vi "外观.vi"(0 "Data In":T9={"启动"=FALSE, "控制命令"=enum."加标回收（启动采配水）", "测量参数"={"氨氮"=TRUE, "总磷"=TRUE, "总氮"=TRUE, "CODMn"=TRUE, "CODCr"=TRUE}} caption="数据输入", 2 "Display State In":T2={"配置信息"={"周期模式"=enum."不启用", "定点周期"={"启动命令"=0, "启动命令 2"=0, "启动命令 3"=0, "启动命令 4"=0, "启动命令 5"=0, "启动命令 6"=0, "启动命令 7"=0, "启动命令 8"=0, "启动命令 9"=0, "启动命令 10"=0, "启动命令 11"=0, "启动命令 12"=0, "启动命令 13"=0, "启动命令 14"=0, "启动命令 15"=0, "启动命令 16"=0, "启动命令 17"=0, "启动命令 18"=0, "启动命令 19"=0, "启动命令 20"=0, "启动命令 21"=0, "启动命令 22"=0, "启动命令 23"=0, "启动命令 24"=0}, "间隔启动"={"启动命令"=0, "启动间隔"=0.0, "启动次数"=0}, "测量参数"={"氨氮"=TRUE, "总磷"=TRUE, "总氮"=TRUE, "CODMn"=TRUE, "CODCr"=TRUE}}, "仪器运行状态"=FALSE, "启动次数"=0, "最近一次启动时间"=timestamp(0 s since 1904-01-01), "最近一次结束时间"=timestamp(0 s since 1904-01-01), "间隔计时"=0.0, "时间源"={"时间源选择"=enum."系统时间源", "外部时间源"=timestamp(0 s since 1904-01-01)}, "引用参数"="", "启用参数"={"氨氮"=TRUE, "总磷"=TRUE, "总氮"=TRUE, "CODMn"=TRUE, "CODCr"=FALSE}} caption="显示状态输入" {"配置信息"."间隔启动"."启动命令" items=["", "加标回收（启动采配水）", "加标回收（不启动采配水）", "水样测试（启动采配水）", "水样测试（不启动采配水）"]; "配置信息"."定点周期"."启动命令 24" items=["", "加标回收（启动采配水）", "加标回收（不启动采配水）", "水样测试（启动采配水）", "水样测试（不启动采配水）"]; "配置信息"."定点周期"."启动命令 23" items=["", "加标回收（启动采配水）", "加标回收（不启动采配水）", "水样测试（启动采配水）", "水样测试（不启动采配水）"]; "配置信息"."定点周期"."启动命令 22" items=["", "加标回收（启动采配水）", "加标回收（不启动采配水）", "水样测试（启动采配水）", "水样测试（不启动采配水）"]; "配置信息"."定点周期"."启动命令 21" items=["", "加标回收（启动采配水）", "加标回收（不启动采配水）", "水样测试（启动采配水）", "水样测试（不启动采配水）"]; "配置信息"."定点周期"."启动命令 20" items=["", "加标回收（启动采配水）", "加标回收（不启动采配水）", "水样测试（启动采配水）", "水样测试（不启动采配水）"]; "配置信息"."定点周期"."启动命令 19" items=["", "加标回收（启动采配水）", "加标回收（不启动采配水）", "水样测试（启动采配水）", "水样测试（不启动采配水）"]; "配置信息"."定点周期"."启动命令 18" items=["", "加标回收（启动采配水）", "加标回收（不启动采配水）", "水样测试（启动采配水）", "水样测试（不启动采配水）"]; "配置信息"."定点周期"."启动命令 17" items=["", "加标回收（启动采配水）", "加标回收（不启动采配水）", "水样测试（启动采配水）", "水样测试（不启动采配水）"]; "配置信息"."定点周期"."启动命令 16" items=["", "加标回收（启动采配水）", "加标回收（不启动采配水）", "水样测试（启动采配水）", "水样测试（不启动采配水）"]; "配置信息"."定点周期"."启动命令 15" items=["", "加标回收（启动采配水）", "加标回收（不启动采配水）", "水样测试（启动采配水）", "水样测试（不启动采配水）"]; "配置信息"."定点周期"."启动命令 14" items=["", "加标回收（启动采配水）", "加标回收（不启动采配水）", "水样测试（启动采配水）", "水样测试（不启动采配水）"]; "配置信息"."定点周期"."启动命令 13" items=["", "加标回收（启动采配水）", "加标回收（不启动采配水）", "水样测试（启动采配水）", "水样测试（不启动采配水）"]; "配置信息"."定点周期"."启动命令 12" items=["", "加标回收（启动采配水）", "加标回收（不启动采配水）", "水样测试（启动采配水）", "水样测试（不启动采配水）"]; "配置信息"."定点周期"."启动命令 11" items=["", "加标回收（启动采配水）", "加标回收（不启动采配水）", "水样测试（启动采配水）", "水样测试（不启动采配水）"]; "配置信息"."定点周期"."启动命令 10" items=["", "加标回收（启动采配水）", "加标回收（不启动采配水）", "水样测试（启动采配水）", "水样测试（不启动采配水）"]; "配置信息"."定点周期"."启动命令 9" items=["", "加标回收（启动采配水）", "加标回收（不启动采配水）", "水样测试（启动采配水）", "水样测试（不启动采配水）"]; "配置信息"."定点周期"."启动命令 8" items=["", "加标回收（启动采配水）", "加标回收（不启动采配水）", "水样测试（启动采配水）", "水样测试（不启动采配水）"]; "配置信息"."定点周期"."启动命令 7" items=["", "加标回收（启动采配水）", "加标回收（不启动采配水）", "水样测试（启动采配水）", "水样测试（不启动采配水）"]; "配置信息"."定点周期"."启动命令 6" items=["", "加标回收（启动采配水）", "加标回收（不启动采配水）", "水样测试（启动采配水）", "水样测试（不启动采配水）"]; "配置信息"."定点周期"."启动命令 5" items=["", "加标回收（启动采配水）", "加标回收（不启动采配水）", "水样测试（启动采配水）", "水样测试（不启动采配水）"]; "配置信息"."定点周期"."启动命令 4" items=["", "加标回收（启动采配水）", "加标回收（不启动采配水）", "水样测试（启动采配水）", "水样测试（不启动采配水）"]; "配置信息"."定点周期"."启动命令 3" items=["", "加标回收（启动采配水）", "加标回收（不启动采配水）", "水样测试（启动采配水）", "水样测试（不启动采配水）"]; "配置信息"."定点周期"."启动命令 2" items=["", "加标回收（启动采配水）", "加标回收（不启动采配水）", "水样测试（启动采配水）", "水样测试（不启动采配水）"]; "配置信息"."定点周期"."启动命令" items=["", "加标回收（启动采配水）", "加标回收（不启动采配水）", "水样测试（启动采配水）", "水样测试（不启动采配水）"]}, 3 "Container State":T8 caption="容器状态") -> (6 "Data Out":T9={"启动"=FALSE, "控制命令"=enum."加标回收（启动采配水）", "测量参数"={"氨氮"=TRUE, "总磷"=TRUE, "总氮"=TRUE, "CODMn"=TRUE, "CODCr"=TRUE}} caption="数据输出", 7 "Display State Out":T2={"配置信息"={"周期模式"=enum."不启用", "定点周期"={"启动命令"=0, "启动命令 2"=0, "启动命令 3"=0, "启动命令 4"=0, "启动命令 5"=0, "启动命令 6"=0, "启动命令 7"=0, "启动命令 8"=0, "启动命令 9"=0, "启动命令 10"=0, "启动命令 11"=0, "启动命令 12"=0, "启动命令 13"=0, "启动命令 14"=0, "启动命令 15"=0, "启动命令 16"=0, "启动命令 17"=0, "启动命令 18"=0, "启动命令 19"=0, "启动命令 20"=0, "启动命令 21"=0, "启动命令 22"=0, "启动命令 23"=0, "启动命令 24"=0}, "间隔启动"={"启动命令"=0, "启动间隔"=0.0, "启动次数"=0}, "测量参数"={"氨氮"=TRUE, "总磷"=TRUE, "总氮"=TRUE, "CODMn"=TRUE, "CODCr"=TRUE}}, "仪器运行状态"=FALSE, "启动次数"=0, "最近一次启动时间"=timestamp(0 s since 1904-01-01), "最近一次结束时间"=timestamp(0 s since 1904-01-01), "间隔计时"=0.0, "时间源"={"时间源选择"=enum."系统时间源", "外部时间源"=timestamp(0 s since 1904-01-01)}, "引用参数"="", "启用参数"={"氨氮"=TRUE, "总磷"=TRUE, "总氮"=TRUE, "CODMn"=TRUE, "CODCr"=FALSE}} caption="显示状态输出" {"配置信息"."间隔启动"."启动命令" items=["", "加标回收（启动采配水）", "加标回收（不启动采配水）", "水样测试（启动采配水）", "水样测试（不启动采配水）"]; "配置信息"."定点周期"."启动命令 24" items=["", "加标回收（启动采配水）", "加标回收（不启动采配水）", "水样测试（启动采配水）", "水样测试（不启动采配水）"]; "配置信息"."定点周期"."启动命令 23" items=["", "加标回收（启动采配水）", "加标回收（不启动采配水）", "水样测试（启动采配水）", "水样测试（不启动采配水）"]; "配置信息"."定点周期"."启动命令 22" items=["", "加标回收（启动采配水）", "加标回收（不启动采配水）", "水样测试（启动采配水）", "水样测试（不启动采配水）"]; "配置信息"."定点周期"."启动命令 21" items=["", "加标回收（启动采配水）", "加标回收（不启动采配水）", "水样测试（启动采配水）", "水样测试（不启动采配水）"]; "配置信息"."定点周期"."启动命令 20" items=["", "加标回收（启动采配水）", "加标回收（不启动采配水）", "水样测试（启动采配水）", "水样测试（不启动采配水）"]; "配置信息"."定点周期"."启动命令 19" items=["", "加标回收（启动采配水）", "加标回收（不启动采配水）", "水样测试（启动采配水）", "水样测试（不启动采配水）"]; "配置信息"."定点周期"."启动命令 18" items=["", "加标回收（启动采配水）", "加标回收（不启动采配水）", "水样测试（启动采配水）", "水样测试（不启动采配水）"]; "配置信息"."定点周期"."启动命令 17" items=["", "加标回收（启动采配水）", "加标回收（不启动采配水）", "水样测试（启动采配水）", "水样测试（不启动采配水）"]; "配置信息"."定点周期"."启动命令 16" items=["", "加标回收（启动采配水）", "加标回收（不启动采配水）", "水样测试（启动采配水）", "水样测试（不启动采配水）"]; "配置信息"."定点周期"."启动命令 15" items=["", "加标回收（启动采配水）", "加标回收（不启动采配水）", "水样测试（启动采配水）", "水样测试（不启动采配水）"]; "配置信息"."定点周期"."启动命令 14" items=["", "加标回收（启动采配水）", "加标回收（不启动采配水）", "水样测试（启动采配水）", "水样测试（不启动采配水）"]; "配置信息"."定点周期"."启动命令 13" items=["", "加标回收（启动采配水）", "加标回收（不启动采配水）", "水样测试（启动采配水）", "水样测试（不启动采配水）"]; "配置信息"."定点周期"."启动命令 12" items=["", "加标回收（启动采配水）", "加标回收（不启动采配水）", "水样测试（启动采配水）", "水样测试（不启动采配水）"]; "配置信息"."定点周期"."启动命令 11" items=["", "加标回收（启动采配水）", "加标回收（不启动采配水）", "水样测试（启动采配水）", "水样测试（不启动采配水）"]; "配置信息"."定点周期"."启动命令 10" items=["", "加标回收（启动采配水）", "加标回收（不启动采配水）", "水样测试（启动采配水）", "水样测试（不启动采配水）"]; "配置信息"."定点周期"."启动命令 9" items=["", "加标回收（启动采配水）", "加标回收（不启动采配水）", "水样测试（启动采配水）", "水样测试（不启动采配水）"]; "配置信息"."定点周期"."启动命令 8" items=["", "加标回收（启动采配水）", "加标回收（不启动采配水）", "水样测试（启动采配水）", "水样测试（不启动采配水）"]; "配置信息"."定点周期"."启动命令 7" items=["", "加标回收（启动采配水）", "加标回收（不启动采配水）", "水样测试（启动采配水）", "水样测试（不启动采配水）"]; "配置信息"."定点周期"."启动命令 6" items=["", "加标回收（启动采配水）", "加标回收（不启动采配水）", "水样测试（启动采配水）", "水样测试（不启动采配水）"]; "配置信息"."定点周期"."启动命令 5" items=["", "加标回收（启动采配水）", "加标回收（不启动采配水）", "水样测试（启动采配水）", "水样测试（不启动采配水）"]; "配置信息"."定点周期"."启动命令 4" items=["", "加标回收（启动采配水）", "加标回收（不启动采配水）", "水样测试（启动采配水）", "水样测试（不启动采配水）"]; "配置信息"."定点周期"."启动命令 3" items=["", "加标回收（启动采配水）", "加标回收（不启动采配水）", "水样测试（启动采配水）", "水样测试（不启动采配水）"]; "配置信息"."定点周期"."启动命令 2" items=["", "加标回收（启动采配水）", "加标回收（不启动采配水）", "水样测试（启动采配水）", "水样测试（不启动采配水）"]; "配置信息"."定点周期"."启动命令" items=["", "加标回收（启动采配水）", "加标回收（不启动采配水）", "水样测试（启动采配水）", "水样测试（不启动采配水）"]}, 8 "Action":T1 caption="动作")   [LabVIEW 2016, in "ZK定时设置.xctl"]
uses:
  <vilib>/_xctls/Container State.ctl
  <vilib>/_xctls/Action.ctl
  <vilib>/Utility/miscctls.llb/LVPositionTypeDef.ctl
  <vilib>/_xctls/XControlSupport.lvlib
  <vilib>/ptbypt/NI_PtbyPt.lvlib
panel:
  in  "周期设置":bool
  # "分钟"
  # "次"
  # "分钟"
  # "次"
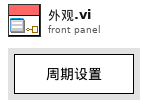
[diagram p1: front panel]
types:
  T1 = typedef "XControlSupport.lvlib/Action.ctl" = cluster{"Data Changed?":bool, "State Changed?":bool, "Action Name":string}
  T2 = typedef "ZK定时设置.xctl/状态.ctl" = cluster{"配置信息":cluster{"周期模式":T3, "定点周期":T4, "间隔启动":T6, "测量参数":T7}, "仪器运行状态":bool, "启动次数":i32, "最近一次启动时间":timestamp, "最近一次结束时间":timestamp, "间隔计时":dbl, "时间源":cluster{"时间源选择":enum16{"系统时间源", "仪器时间源"}, "外部时间源":timestamp}, "引用参数":string, "启用参数":T7}
  T3 = typedef "ZK定时设置.xctl/周期模式设置.ctl" = enum16{"不启用", "定点模式", "间隔模式"}
  T4 = typedef "ZK定时设置.xctl/定点周期设置.ctl" = cluster{"启动命令":T5, "启动命令 2":T5, "启动命令 3":T5, "启动命令 4":T5, "启动命令 5":T5, "启动命令 6":T5, "启动命令 7":T5, "启动命令 8":T5, "启动命令 9":T5, "启动命令 10":T5, "启动命令 11":T5, "启动命令 12":T5, "启动命令 13":T5, "启动命令 14":T5, "启动命令 15":T5, "启动命令 16":T5, "启动命令 17":T5, "启动命令 18":T5, "启动命令 19":T5, "启动命令 20":T5, "启动命令 21":T5, "启动命令 22":T5, "启动命令 23":T5, "启动命令 24":T5}
  T5 = typedef "ZK定时设置.xctl/启动命令选择.ctl" = u16
  T6 = typedef "ZK定时设置.xctl/间隔启动设置.ctl" = cluster{"启动命令":T5, "启动间隔":dbl, "启动次数":i32}
  T7 = typedef "ZK定时设置.xctl/测量参数.ctl" = cluster{"氨氮":bool, "总磷":bool, "总氮":bool, "CODMn":bool, "CODCr":bool}
  T8 = typedef "XControlSupport.lvlib/Container State.ctl" = cluster{"Indicator?":bool, "Run Mode?":bool, " Refnum":refnum<vi>}
  T9 = typedef "ZK定时设置.xctl/数据.ctl" = cluster{"启动":bool, "控制命令":T10, "测量参数":T7}
  T10 = typedef "ZK定时设置.xctl/国标控制命令.ctl" = enum16{"加标回收（启动采配水）", "加标回收（不启动采配水）", "水样测试（启动采配水）", "水样测试（不启动采配水）"}
  T11 = typedef "LVPositionTypeDef.ctl" = cluster{"Left":i32, "Top":i32}
  T12 = cluster{"周期模式":T3, "定点周期":T4, "间隔设置":cluster{"启动命令":T5, "启动间隔":dbl, "启动次数":i32}, "测量参数":T7}
  T13 = cluster{"周期模式":T3, "定点周期":T4, "间隔启动":T6, "测量参数":T7}
  T14 = cluster{"时间源选择":enum16{"系统时间源", "仪器时间源"}, "外部时间源":timestamp}
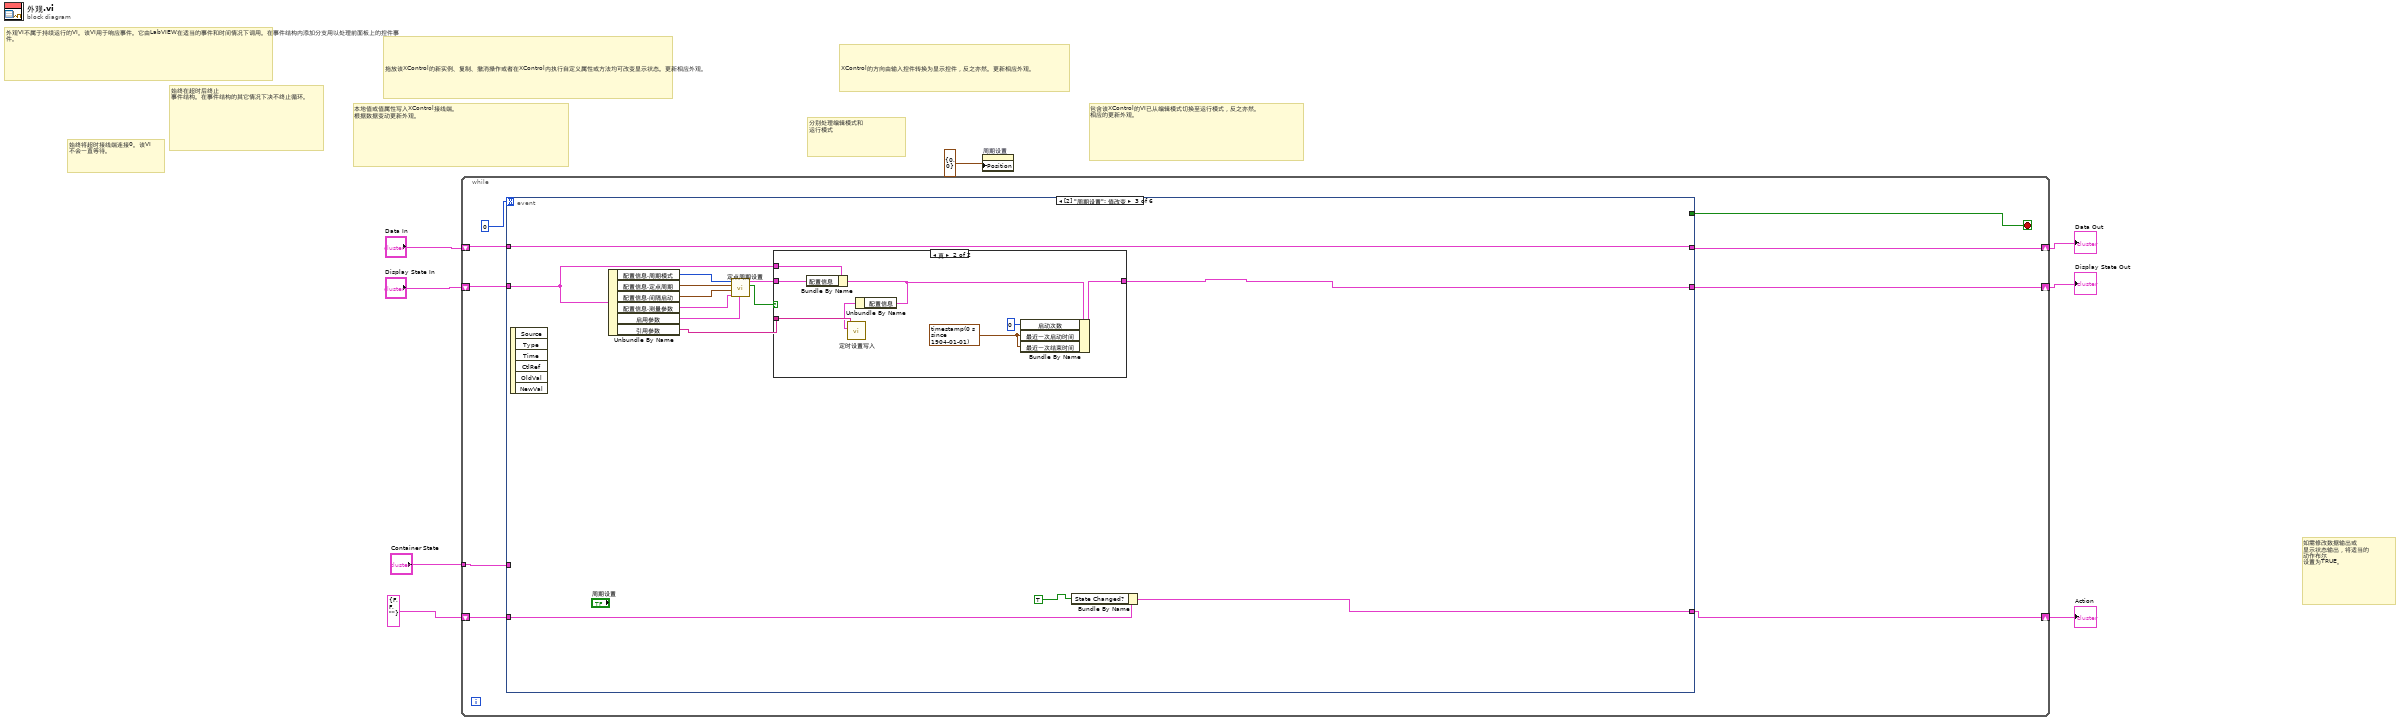
[diagram p0: block diagram]
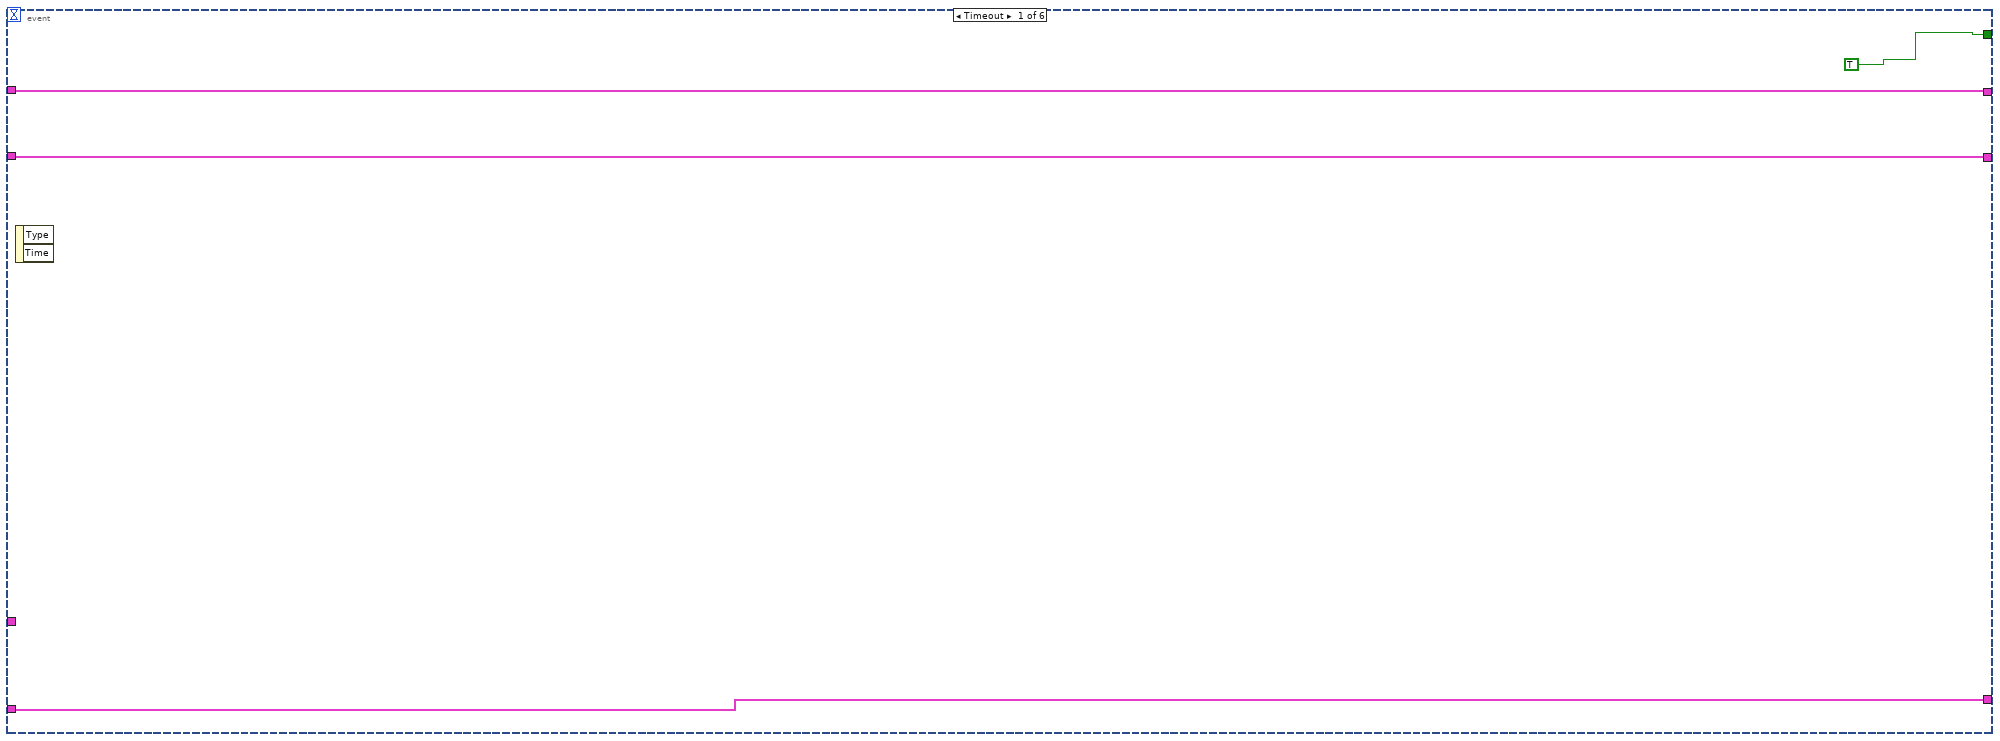
[diagram p2: hidden frame]
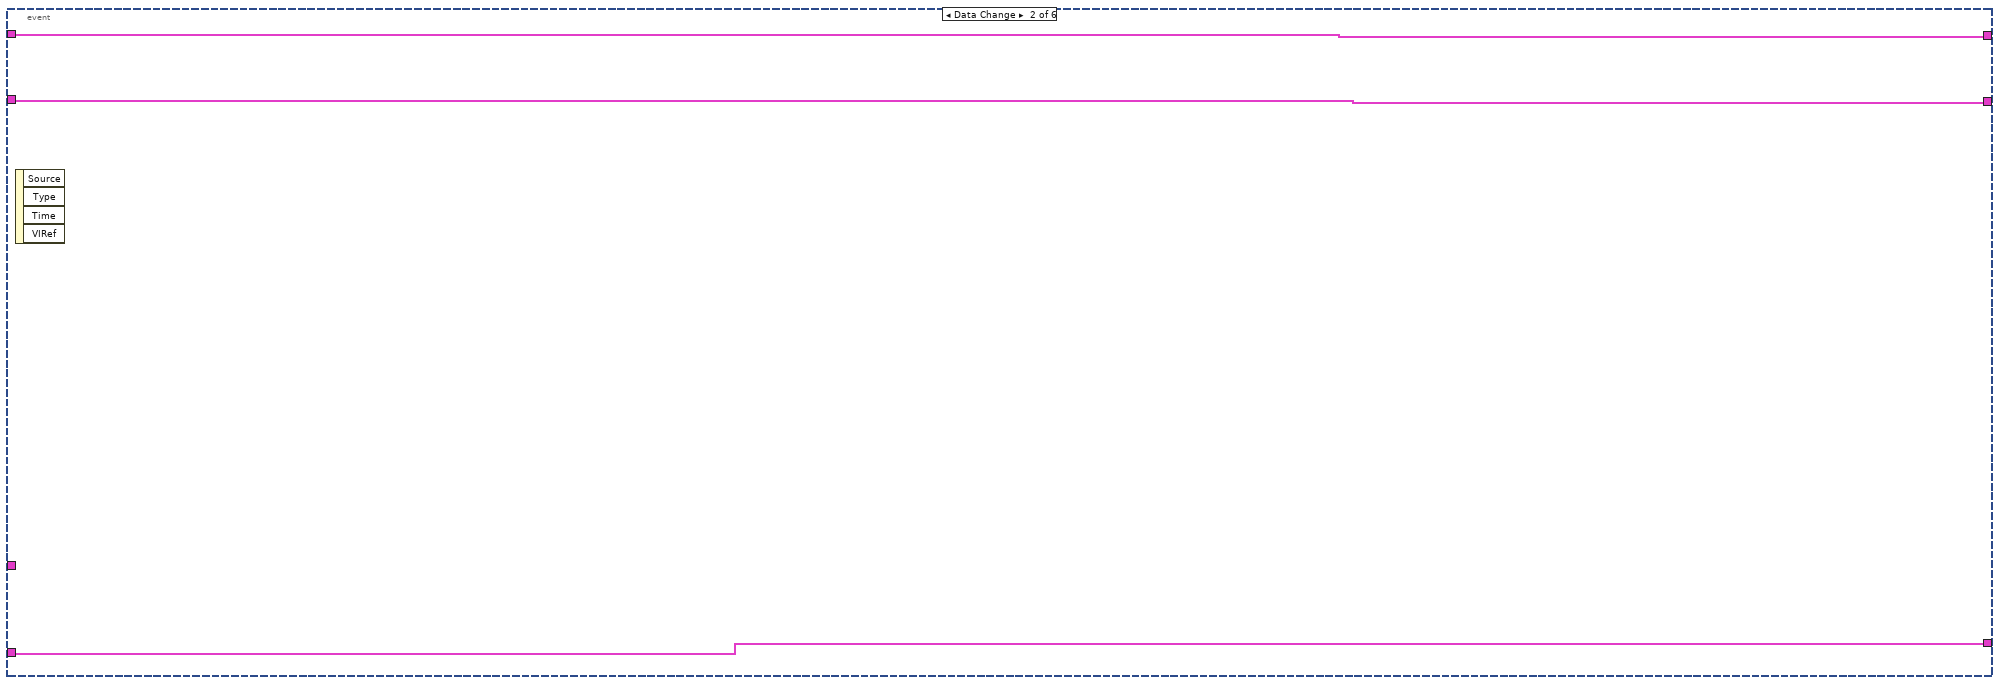
[diagram p3: hidden frame]
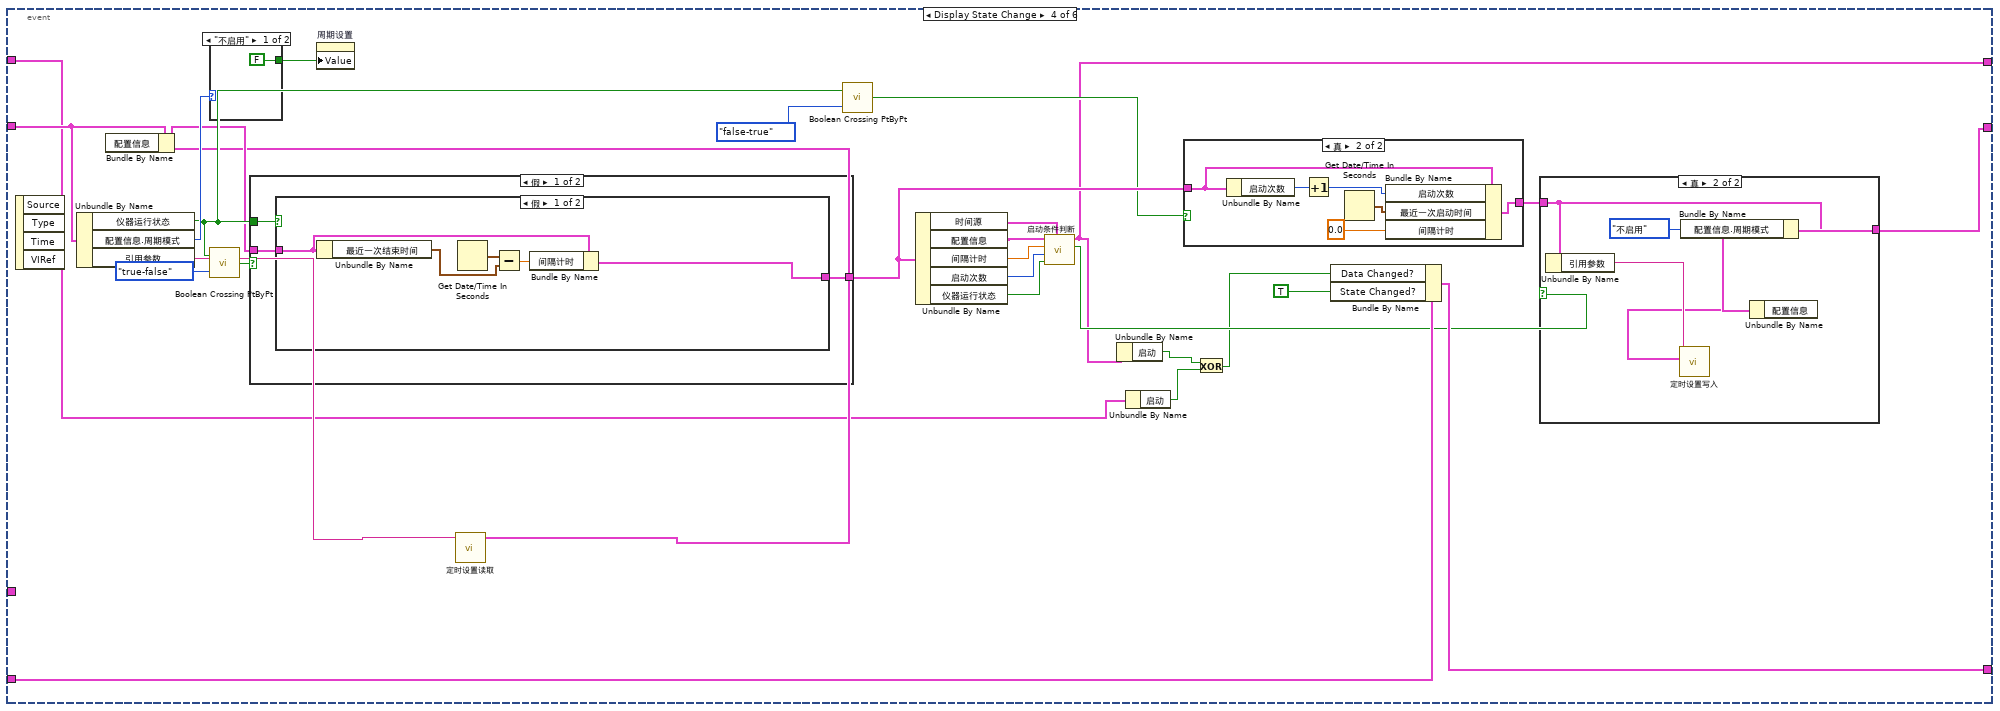
[diagram p5: hidden frame]
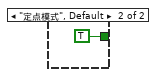
[diagram p7: hidden frame]
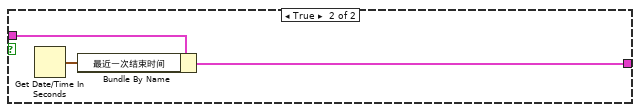
[diagram p9: hidden frame]
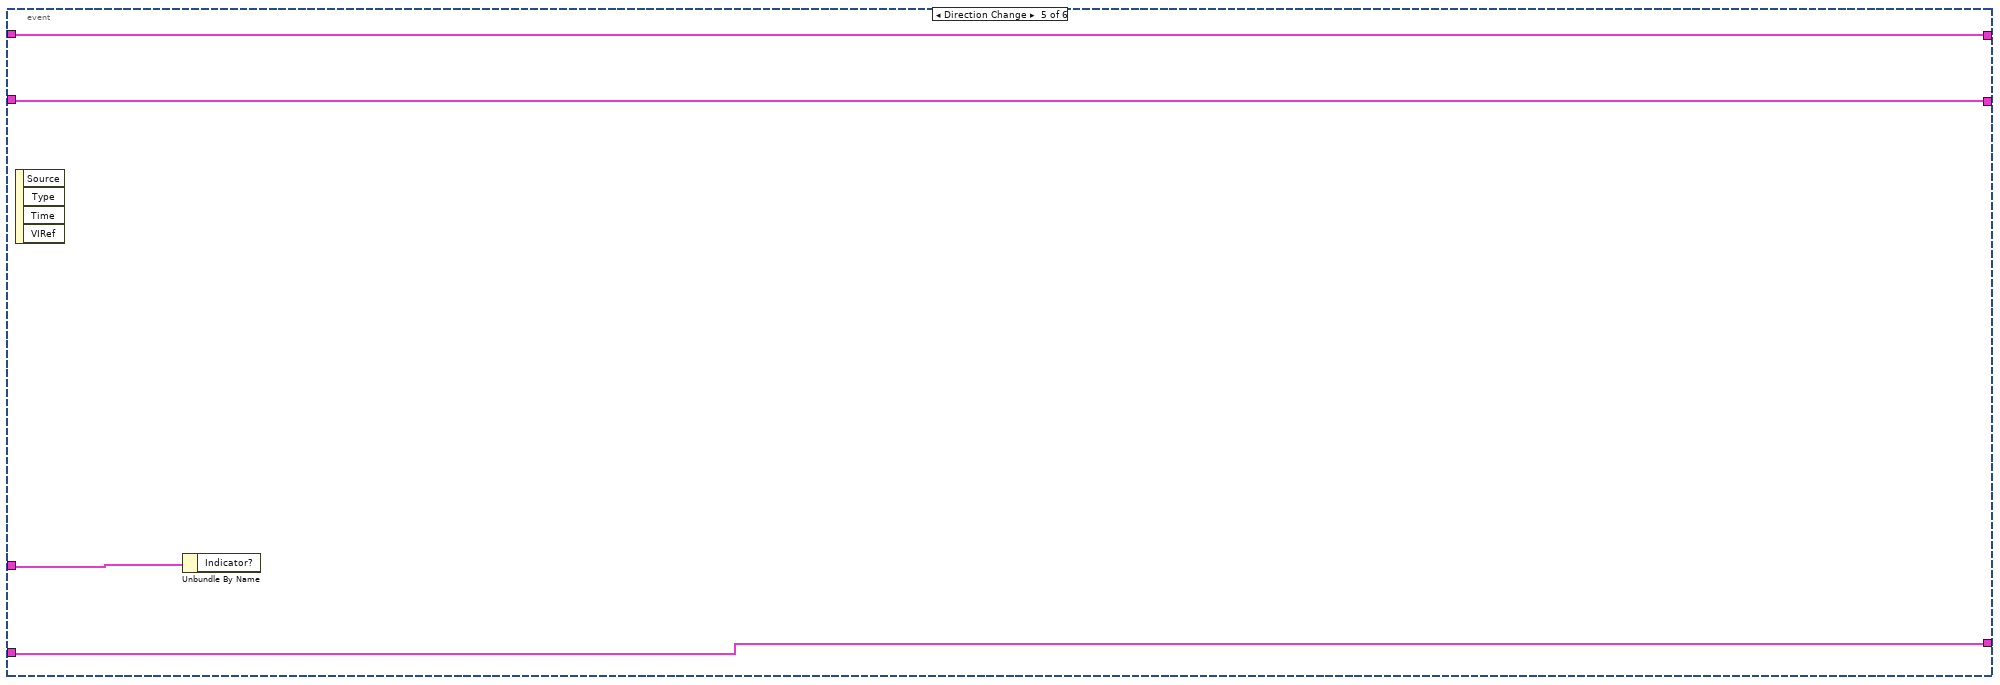
[diagram p11: hidden frame]
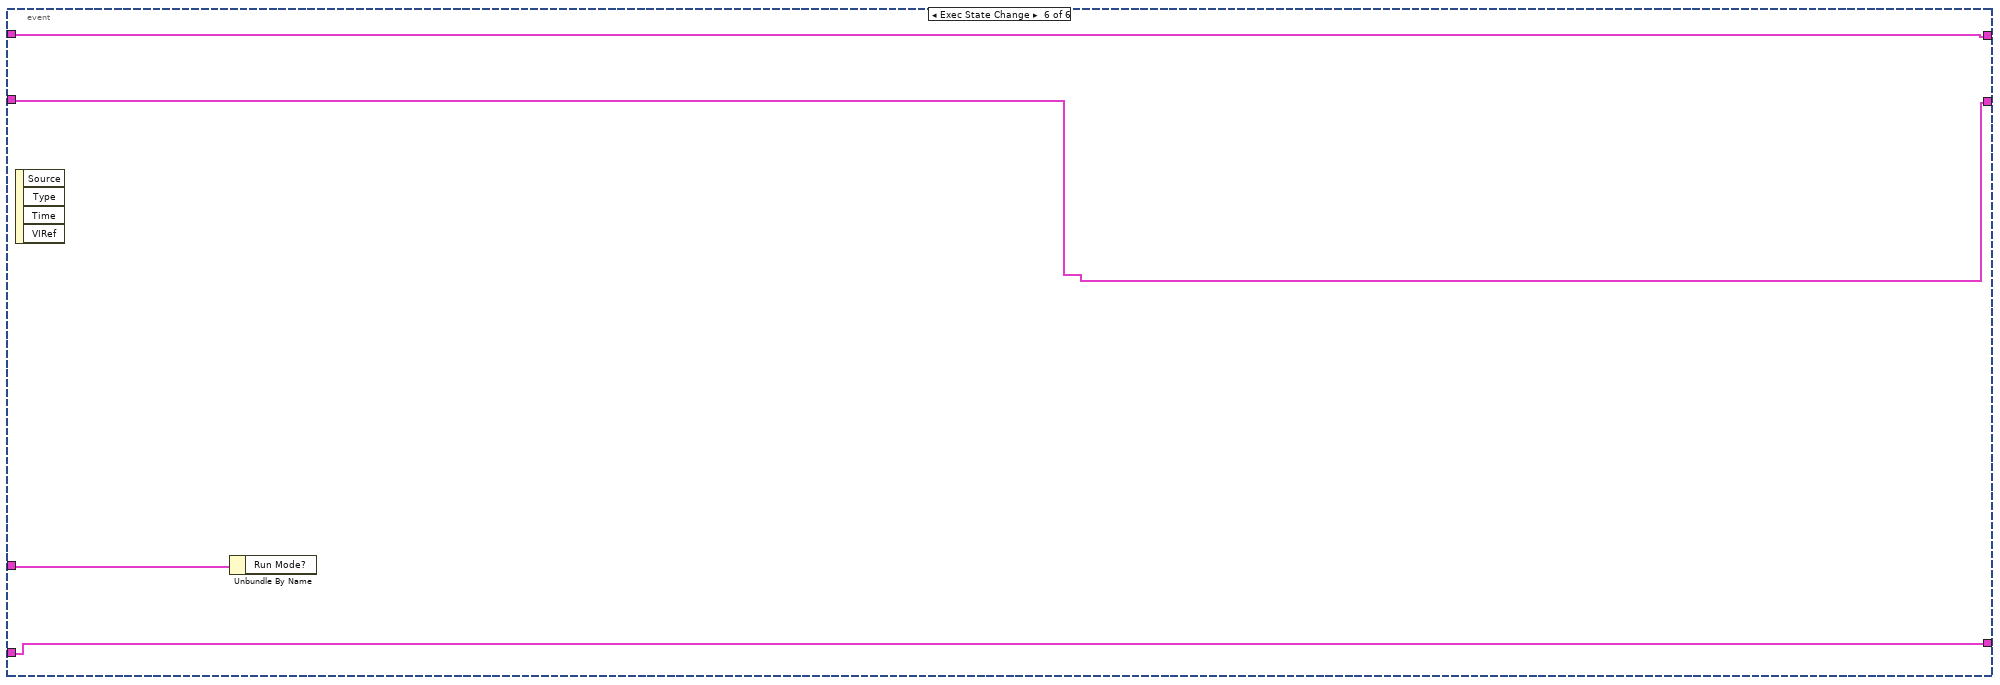
[diagram p12: hidden frame]
diagram:
  # "分别处理编辑模式和\n运行模式"
  # "包含该XControl的VI已从编辑模式切换至运行模式，反之亦然。\n相应的更新外观。"
  # "XControl的方向由输入控件转换为显示控件，反之亦然。更新相应外观。"
  # "始终将超时接线端连接0。该VI\n不会一直等待。"
  # "拖放该XControl的新实例、复制、撤消操作或者在XControl内执行自定义属性或方法均可改变显示状态。更新相应外观。"
  # "本地值或值属性写入XControl接线端。\n根据数据变动更新外观。"
  # "始终在超时后终止\n事件结构。在事件结构的其它情况下决不终止循环。"
  # "外观VI不属于持续运行的VI。该VI用于响应事件。它由LabVIEW在适当的事件和时间情况下调用。在事件结构内添加分支用以处理前面板上的控件事件。"
  # "如需修改数据输出或\n显示状态输出，将适当的\n动作布尔\n设置为TRUE。"
  n1 = while {
    shift-right: [w16] -> w5
    shift-left: "Display State In" -> [w17]
    tunnel: "Container State" -> [w13]
    shift-right: [w11] -> w8
    shift-left: "Data In" -> [w12]
    shift-right: [w9] -> w3
    shift-left: T1 {"Data Changed?"=FALSE, "State Changed?"=FALSE, "Action Name"=""} ("Action") -> [w10]
    stop <- w15 stop-if-true
    n2 = event shown="[2] \"周期设置\": 值改变" {
      selector: _ -> [_ _ _ _ _ _]
      dyn-events: _ -> [_ _ _ _ _ _]
      timeout: 0 -> [_ _ _ _ _ _]
      tunnel: w17 -> [w19 w23 w35 w70 w105 w107]
      tunnel: [w19 w23 w28 w60 w105 w107] -> w16
      tunnel: [TRUE _ _ _ _ _] -> w15
      tunnel: w13 -> [_ _ _ _ w106 w110]
      tunnel: w12 -> [w18 w24 w36 w51 w104 w108]
      tunnel: [w18 w24 w36 w52 w104 w108] -> w11
      tunnel: [w20 w22 w33 w73 w103 w109] -> w9
      tunnel: w10 -> [w20 w22 w34 w74 w103 w109]
      event Timeout {
        n3 = event-data() -> ()  [unwired: 1 in, 2 out]
      }
      event Data Change {
        n4 = event-data() -> ()  [unwired: 1 in, 4 out]
      }
      event "周期设置": Value Change {
        n5 = event-data() -> ()  [unwired: 1 in, 6 out]
        n6 = Unbundle By Name(w35) -> ("配置信息.周期模式"=w30:T3, "配置信息.定点周期"=w37:T4, "配置信息.间隔启动"=w38:T6, "配置信息.测量参数"=w27:T7, "启用参数"=w25:T7, "引用参数"=w26:string)
        n7 = call "定点周期设置.vi"("启用参数"=w25, "测量参数"=w27, "间隔启动"=w38, "定点周期"=w37, "周期模式"=w30) -> ("保存输出"=w29:bool, "周期设置输出"=w31:T12)  [unwired: 5 in]
        n8 = case shown="真" w29 {
          tunnel: w35 -> [w39 w47]
          tunnel: [w39 w46] -> w28
          tunnel: w31 -> [_ w42]
          tunnel: w26 -> [_ w43]
          frame False {
          }
          frame True {
            w45 = timestamp(0 s since 1904-01-01) ("最近一次启动时间")
            n9 = Bundle By Name(cluster=w47, "配置信息"=w42) -> (w41:T2)
            n10 = Unbundle By Name(w41) -> ("配置信息"=w40:T13)
            n11 = call "定时设置写入.vi"("INI Fomatted Cluster"=w40, "测试参数"=w43) -> ()  [unwired: 10 in]
            n12 = Bundle By Name(cluster=w41, "启动次数"=0, "最近一次启动时间"=w45, "最近一次结束时间"=w45) -> (w46:T2)
          }
        }
        n13 = Bundle By Name(cluster=w34, "State Changed?"=TRUE) -> (w33:T1)
      }
      event Display State Change {
        n14 = event-data() -> ()  [unwired: 1 in, 4 out]
        n15 = Unbundle By Name(w70) -> ("仪器运行状态"=w58:bool, "配置信息.周期模式"=w64:T3, "引用参数"=w55:string)
        n16 = case shown="\"不启用\"" w64 {
          tunnel: [FALSE TRUE] -> w63
          frame "不启用" {
          }
          frame "定点模式", Default {
          }
        }
        n17 = call <vilib>:"Boolean Crossing PtByPt.vi"("direction"=enum16{"either", "false-true", "true-false"}."true-false", "input"=w58) -> ("crossing"=w71:bool)  [unwired: 1 in]
        n18 = property on="周期设置" class="Bool (严格)"("Value"=w63) -> ()  [unwired: 2 in, 2 out]
        n19 = call "定时设置读取.vi"("引用参数"=w55) -> ("周期设置输出"=w53:T13)  [unwired: 10 in]
        n20 = Bundle By Name(cluster=w70, "配置信息"=w53) -> (w54:T2)
        n21 = case shown="假" w71 {
          tunnel: w54 -> [w86 w95]
          tunnel: [w85 w94] -> w69
          tunnel: w58 -> [w84 _]
          frame False {
            n22 = case shown="假" w84 {
              tunnel: w86 -> [w90 w92]
              tunnel: [w88 w92] -> w85
              frame False {
                n23 = Unbundle By Name(w90) -> ("最近一次结束时间"=w87:timestamp)
                n24 = Get Date/Time In Seconds() -> (seconds since 1Jan1904=w91:timestamp)
                n25 = Subtract(x=w91, y=w87) -> (x-y=w89:dbl)
                n26 = Bundle By Name(cluster=w90, "间隔计时"=w89) -> (w88:T2)
              }
              frame True {
              }
            }
          }
          frame True {
            n27 = Get Date/Time In Seconds() -> (seconds since 1Jan1904=w93:timestamp)
            n28 = Bundle By Name(cluster=w95, "最近一次结束时间"=w93) -> (w94:T2)
          }
        }
        n29 = call <vilib>:"Boolean Crossing PtByPt.vi"("direction"=enum16{"either", "false-true", "true-false"}."false-true", "input"=w58) -> ("crossing"=w57:bool)  [unwired: 1 in]
        n30 = Unbundle By Name(w69) -> ("时间源"=w56:T14, "配置信息"=w68:T13, "间隔计时"=w67:dbl, "启动次数"=w66:i32, "仪器运行状态"=w65:bool)
        n31 = call "启动条件判断.vi"("时间源"=w56, "仪器状态"=w65, "启动次数"=w66, "间隔计时"=w67, "周期设置输出"=w68) -> ("重新配置"=w61:bool, "Data"=w52:T9)  [unwired: 5 in]
        n32 = Unbundle By Name(w52) -> ("启动"=w49:bool)
        n33 = Unbundle By Name(w51) -> ("启动"=w50:bool)
        n34 = case shown="真" w57 {
          tunnel: w69 -> [w96 w100]
          tunnel: [w96 w102] -> w62
          frame False {
          }
          frame True {
            n35 = Unbundle By Name(w100) -> ("启动次数"=w99:i32)
            n36 = Increment(x=w99) -> (x+1=w98:i32)
            n37 = Get Date/Time In Seconds() -> (seconds since 1Jan1904=w101:timestamp)
            n38 = Bundle By Name(cluster=w100, "启动次数"=w98, "最近一次启动时间"=w101, "间隔计时"=0.0) -> (w102:T2)
          }
        }
        n39 = Exclusive Or(1:w50, 2:w49) -> (0:w48:bool)
        n40 = Bundle By Name(cluster=w74, "Data Changed?"=w48, "State Changed?"=TRUE) -> (w73:T1)
        n41 = case shown="真" w61 {
          tunnel: w62 -> [w76 w79]
          tunnel: [w76 w80] -> w60
          frame False {
          }
          frame True {
            n42 = Unbundle By Name(w79) -> ("引用参数"=w78:string)
            n43 = Bundle By Name(cluster=w79, "配置信息.周期模式"=周期模式设置."不启用") -> (w80:T2)
            n44 = Unbundle By Name(w80) -> ("配置信息"=w77:T13)
            n45 = call "定时设置写入.vi"("INI Fomatted Cluster"=w77, "测试参数"=w78) -> ()  [unwired: 10 in]
          }
        }
      }
      event Direction Change {
        n46 = event-data() -> ()  [unwired: 1 in, 4 out]
        n47 = Unbundle By Name(w106) -> ()  [unwired: 1 out]
      }
      event Exec State Change {
        n48 = event-data() -> ()  [unwired: 1 in, 4 out]
        n49 = Unbundle By Name(w110) -> ()  [unwired: 1 out]
      }
    }
  }
  "Display State Out" <- w5
  "Data Out" <- w8
  "Action" <- w3
  n50 = property on="周期设置" class="Bool (严格)"("Position"=T11 {"Left"=0, "Top"=0} ("位置")) -> ()  [unwired: 2 in, 2 out]
